vi "dosimat_fill.vi"(2 "error in":errorcluster, 3 "Dosimat Port In":refnum<visa-resource-name>="COM1") -> (0 "error out":errorcluster, 1 "Dosimat Port Out":refnum<visa-resource-name>="COM1")   [LabVIEW 2010]
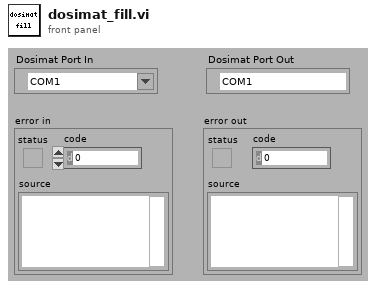
[diagram p1: front panel]
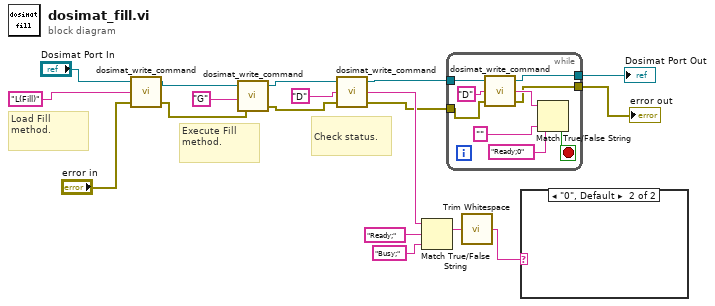
[diagram p0: block diagram]
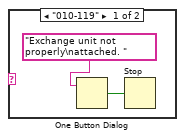
[diagram p2: hidden frame]
diagram:
  # "Check status."
  # "Execute Fill method."
  # "Load Fill method."
  n1 = call "dosimat_write_command.vi"("error in"="error in", "write buffer"="L(Fill)", "Dosimat Port In"="Dosimat Port In") -> ("error out"=w13:errorcluster, "Dosimat Port Out"=w14:refnum<visa-resource-name>)  [unwired: 1 out]
  n2 = call "dosimat_write_command.vi"("error in"=w13, "write buffer"="G", "Dosimat Port In"=w14) -> ("error out"=w5:errorcluster, "Dosimat Port Out"=w6:refnum<visa-resource-name>)  [unwired: 1 out]
  n3 = call "dosimat_write_command.vi"("error in"=w5, "write buffer"="D", "Dosimat Port In"=w6) -> ("error out"=w3:errorcluster, "read buffer"=w10:string, "Dosimat Port Out"=w4:refnum<visa-resource-name>)
  n4 = Match True/False String(2:"Busy;" ("false string"), 3:"Ready;" ("true string"), 4:w10) -> (1:w8:string)  [unwired: 1 out]
  n5 = while {
    tunnel: w4 -> [w22]
    tunnel: w3 -> [w21]
    tunnel: [w20] -> w2
    tunnel: [w19] -> w1
    stop <- w25 stop-if-true
    n6 = call "dosimat_write_command.vi"("error in"=w21, "write buffer"="D", "Dosimat Port In"=w22) -> ("error out"=w19:errorcluster, "read buffer"=w23:string, "Dosimat Port Out"=w20:refnum<visa-resource-name>)
    n7 = Match True/False String(2:"" ("false string"), 3:"Ready;0" ("true string"), 4:w23) -> (0:w25:bool)  [unwired: 1 out]
  }
  "error out" <- w1
  "Dosimat Port Out" <- w2
  n8 = call <vilib>:"Trim Whitespace.vi"("string"=w8) -> ("trimmed string"=w7:string)  [unwired: 1 in]
  n9 = case shown="\"0\", Default" w7 {
    frame "010-119" {
      n10 = One Button Dialog(message="Exchange unit not properly\nattached. ") -> (true=w28:bool)  [unwired: 1 in]
      n11 = Stop(stop? (T)=w28) -> ()
    }
    frame "0", Default {
    }
  }
